vi "Get Wavelength Setting State.vi"(1 "Channel":i32=1) -> (0 "Wavelength Setting State":string)   [LabVIEW 2020]
panel:
  out "body":string
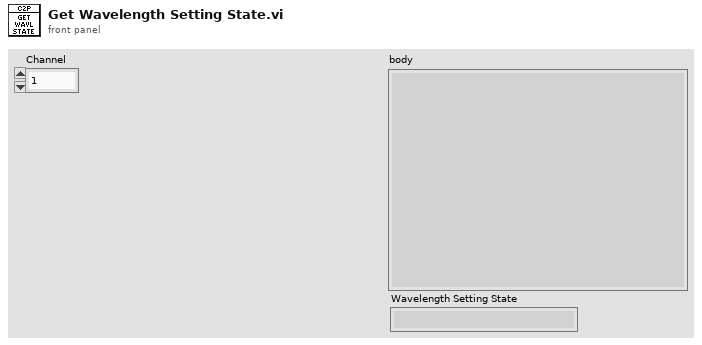
[diagram p1: front panel]
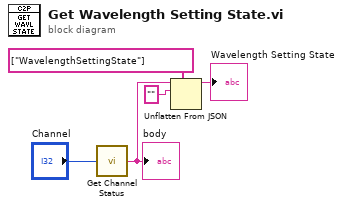
[diagram p0: block diagram]
diagram:
  n1 = call "Get Channel Status.vi"("Channel"="Channel") -> ("body"=w2:string)
  "body" <- w2
  n2 = Unflatten From JSON(path=string[] ["WavelengthSettingState"], JSON string=w2, type and defaults="") -> (value=→"Wavelength Setting State":string)  [unwired: 4 in, 1 out]
